vi "tm_getparameterlimits_40.vi"(7 "Reconfigure (F)":bool, 8 "error in (no error)":errorcluster, 10 "Parameter":u32(ring)=4215968 items=["SENSOR MODE"=4212128, "SENSOR MODE LINE BUNDLE HEIGHT"=4212192, "READOUT DIRECTION"=4211904, "BIT PER CHANNEL"=4342976, "EXPOSURE TIME"=2049184, "CONTRAST GAIN"=3163312, "BINNING"=4215968, "TIMING READOUT TIME"=4223904, "INTERNAL FRAME RATE"=4225952, "INTERNAL FRAME INTERVAL"=4225968, "INTERNAL LINE SPEED"=4226000, "IMAGE WIDTH"=4343200, "IMAGE HEIGHT"=4343216, "IMAGE ROWBYTES"=4343232, "IMAGE FRAMEBYTES"=4343248, "IMAGE PIXEL TYPE"=4343296], 11 "Handle in":u32) -> (0 "error out":errorcluster, 1 "default":dbl, 2 "Range":cluster{"min":dbl, "max":dbl, "step":dbl}, 3 "Handle out":u32, 4 "Value Names":cluster{"Name":string, "Value":dbl}[](array[cluster]), 5 "Writable":bool, 6 "Text Values":bool)   [LabVIEW 2023]
uses:
  tmcamcon.dll
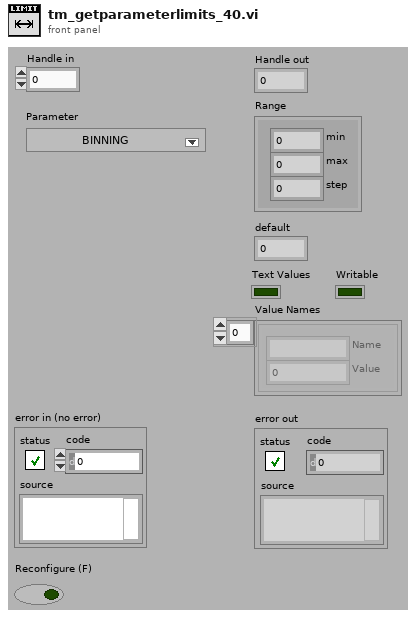
[diagram p1: front panel]
types:
  T1 = cluster{"Property Name":string, "Property ID":i32}[]
  T2 = cluster{"Property Name":string, "Property ID":i32}
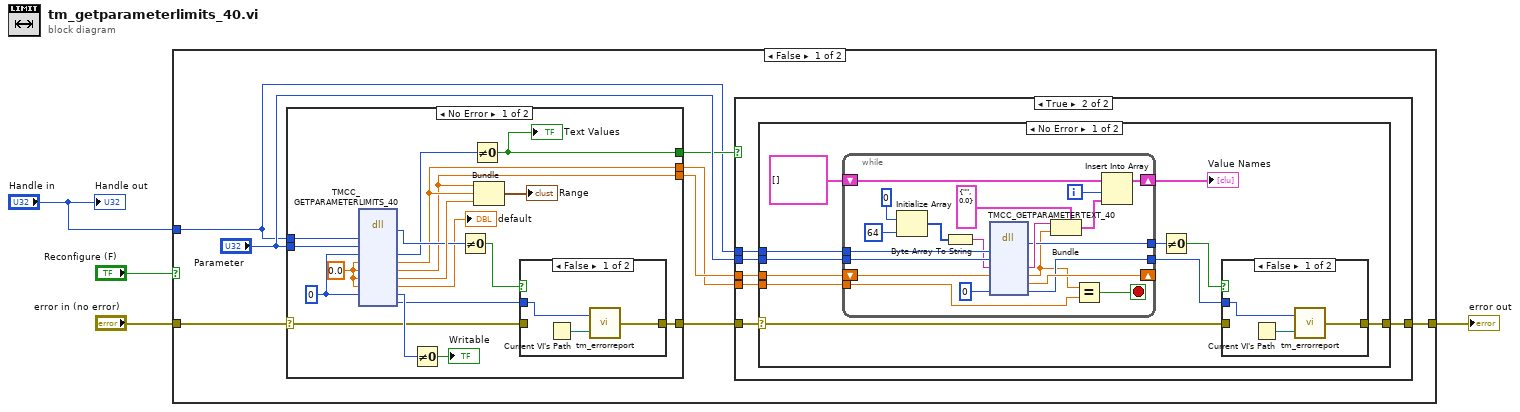
[diagram p0: block diagram]
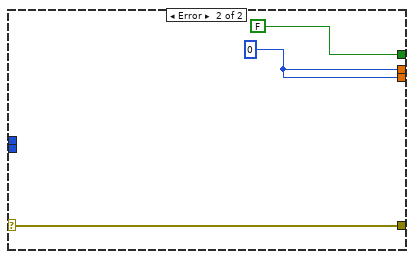
[diagram p6: hidden frame]
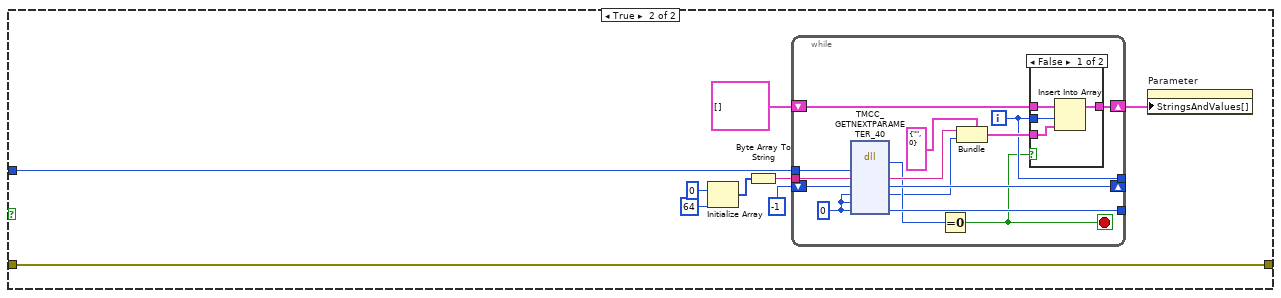
[diagram p7: hidden frame]
diagram:
  n1 = case shown="False" "Reconfigure (F)" {
    tunnel: "error in (no error)" -> [w6 w89]
    tunnel: [w7 w89] -> w3
    tunnel: "Handle in" -> [w5 w81]
    frame False {
      n2 = case shown="No Error" w6 {
        selector: w6 -> [w59 w80]
        tunnel: [w56 w80] -> w9
        tunnel: "Parameter" -> [w73 _]
        tunnel: w5 -> [w67 _]
        tunnel: [w65 w78] -> w10
        tunnel: [w64 w78] -> w11
        tunnel: [w66 FALSE] -> w8
        frame No Error {
          w72 = 0.0
          w60 = u32 0
          n3 = dll-call lib="tmcamcon.dll" fn="TMCC_GETPARAMETERLIMITS_40"("HDCAM"=w67, "propertyid"=w73, "text"=w60, "max"=w72, "min"=w72, "step"=w72, "default"=w72, "writable"=w60) -> ("return type"=w69:u32, "text"=w68:u32, "max"=w65:dbl, "min"=w64:dbl, "step"=w70:dbl, "default"=→"default":dbl, "writable"=w61:u32, "Erval"=w58:i32)  [unwired: 6 in, 2 out]
          n4 = Not Equal To 0?(x=w61) -> (x != 0?=→"Writable":bool)
          n5 = Not Equal To 0?(x=w69) -> (x != 0?=w57:bool)
          n6 = Not Equal To 0?(x=w68) -> (x != 0?=w66:bool)
          "Text Values" <- w66
          n7 = Bundle("min"=w64, "max"=w65, "step"=w70) -> (→"Range":cluster{"min":dbl, "max":dbl, "step":dbl})  [unwired: 1 in]
          n8 = case shown="False" w57 {
            tunnel: w59 -> [_ w77]
            tunnel: [w75 w77] -> w56
            tunnel: w58 -> [w74 _]
            frame False {
              n9 = Current VI's Path() -> (path=w76:path)
              n10 = call "tm_errorreport.vi"("Source"=w76, "Error"=w74) -> ("error out"=w75:errorcluster)
            }
            frame True {
            }
          }
        }
        frame Error {
          w78 = 0
        }
      }
      n11 = case shown="True" w8 {
        tunnel: w9 -> [w13 w19]
        tunnel: w5 -> [_ w18]
        tunnel: "Parameter" -> [_ w17]
        tunnel: w11 -> [_ w16]
        tunnel: w10 -> [_ w15]
        tunnel: [w13 w14] -> w7
        frame False {
        }
        frame True {
          n12 = case shown="No Error" w19 {
            selector: w19 -> [w23 w55]
            tunnel: [w20 w55] -> w14
            tunnel: w18 -> [w27 _]
            tunnel: w17 -> [w26 _]
            tunnel: w16 -> [w25 _]
            tunnel: w15 -> [w24 _]
            frame No Error {
              n13 = while {
                shift-right: [w53] -> w29
                shift-left: cluster{"Name":string, "Value":dbl}[] [] ("Value Names") -> [w54]
                tunnel: [w50] -> w28
                tunnel: w27 -> [w48]
                tunnel: w26 -> [w47]
                shift-right: [w45] -> _
                shift-left: w25 -> [w46]
                tunnel: [w42] -> w22
                tunnel: w24 -> [w41]
                i -> [w49]
                stop <- w39 stop-if-true
                n14 = Initialize Array(u8 0, 64) -> (w36:u8[])
                n15 = Byte Array To String(unsigned byte array=w36) -> (string=w35:string)
                n16 = dll-call lib="tmcamcon.dll" fn="TMCC_GETPARAMETERTEXT_40"("HDCAM"=w48, "propertyid"=w47, "name"=w35, "value"=w46, "Erval"=0) -> ("return type"=w50:u32, "name"=w51:string, "value"=w40:dbl, "nextvalue"=w45:dbl, "Erval"=w42:i32)  [unwired: 6 in, 2 out]
                n17 = Bundle(cluster=cluster{"name":string, "value":dbl} {"name"="", "value"=0.0}, "name"=w51, "value"=w40) -> (w52:cluster{"name":string, "value":dbl})
                n18 = Equal?(x=w40, y=w41) -> (x = y?=w39:bool)
                n19 = Insert Into Array(array=w54, index=w49, new element=w52) -> (w53:cluster{"Name":string, "Value":dbl}[])
              }
              "Value Names" <- w29
              n20 = Not Equal To 0?(x=w28) -> (x != 0?=w21:bool)
              n21 = case shown="False" w21 {
                tunnel: w23 -> [_ w34]
                tunnel: [w32 w34] -> w20
                tunnel: w22 -> [w31 _]
                frame False {
                  n22 = Current VI's Path() -> (path=w33:path)
                  n23 = call "tm_errorreport.vi"("Source"=w33, "Error"=w31) -> ("error out"=w32:errorcluster)
                }
                frame True {
                }
              }
            }
            frame Error {
            }
          }
        }
      }
    }
    frame True {
      n24 = Initialize Array(u8 0 ("element"), 64 ("dimension size")) -> (w87:u8[])
      n25 = Byte Array To String(unsigned byte array=w87) -> (string=w84:string)
      n26 = while {
        shift-right: [w103] -> w82
        shift-left: T1 [] ("Array") -> [w104]
        tunnel: [w99] -> _
        tunnel: [w97] -> _
        tunnel: w84 -> [w96]
        tunnel: w81 -> [w95]
        shift-right: [w98] -> _
        shift-left: -1 ("func_num") -> [w100]
        i -> [w97]
        stop <- w93 stop-if-true
        w90 = 0 ("option")
        n27 = dll-call lib="tmcamcon.dll" fn="TMCC_GETNEXTPARAMETER_40"("HDCAM"=w95, "name"=w96, "func_num"=w100, "func_id"=w90, "option"=w90, "Erval"=w90) -> ("return type"=w92:u32, "name"=w101:string, "func_num"=w98:i32, "func_id"=w91:i32, "Erval"=w99:i32)  [unwired: 5 in, 2 out]
        n28 = Equal To 0?(x=w92) -> (x = 0?=w93:bool)
        n29 = Bundle(cluster=T2 {"Property Name"="", "Property ID"=0} ("new element/subarray"), "Property Name"=w101, "Property ID"=w91) -> (w102:T2)
        n30 = case shown="False" w93 {
          tunnel: w104 -> [w108 w109]
          tunnel: [w107 w109] -> w103
          tunnel: w97 -> [w106 _]
          tunnel: w102 -> [w105 _]
          frame False {
            n31 = Insert Into Array(array=w108, index=w106, new element=w105) -> (w107:T1)
          }
          frame True {
          }
        }
      }
      n32 = property on="Parameter" class="Ring (strict)"("StringsAndValues[]"=w82) -> ()  [unwired: 2 in, 2 out]
    }
  }
  "error out" <- w3
  "Handle out" <- "Handle in"
